vi "need_to_update_settings.vi"(1 "previous settings value cluster":T1, 2 "settings value cluster":T1) -> (0 "New Settings Exist?":bool)   [LabVIEW 2015]
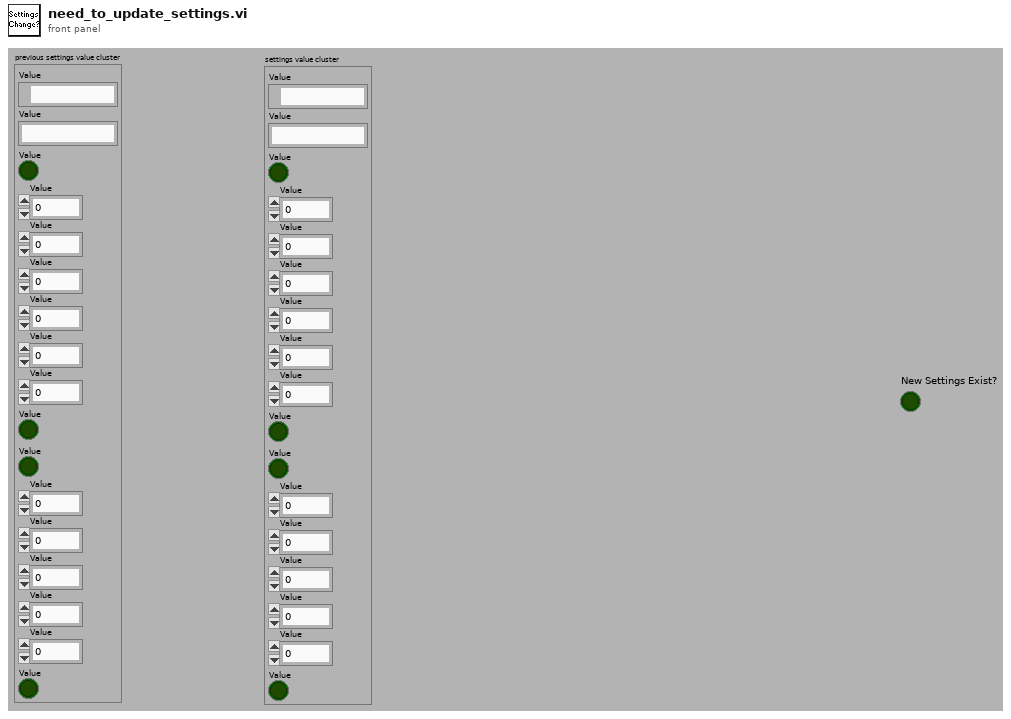
[diagram p1: front panel]
types:
  T1 = cluster{"Value":path, "Value":string, "Value":bool, "Value":dbl, "Value":dbl, "Value":i32, "Value":i32, "Value":dbl, "Value":u16, "Value":bool, "Value":bool, "Value":i32, "Value":i32, "Value":i32, "Value":u32, "Value":i32, "Value":bool}
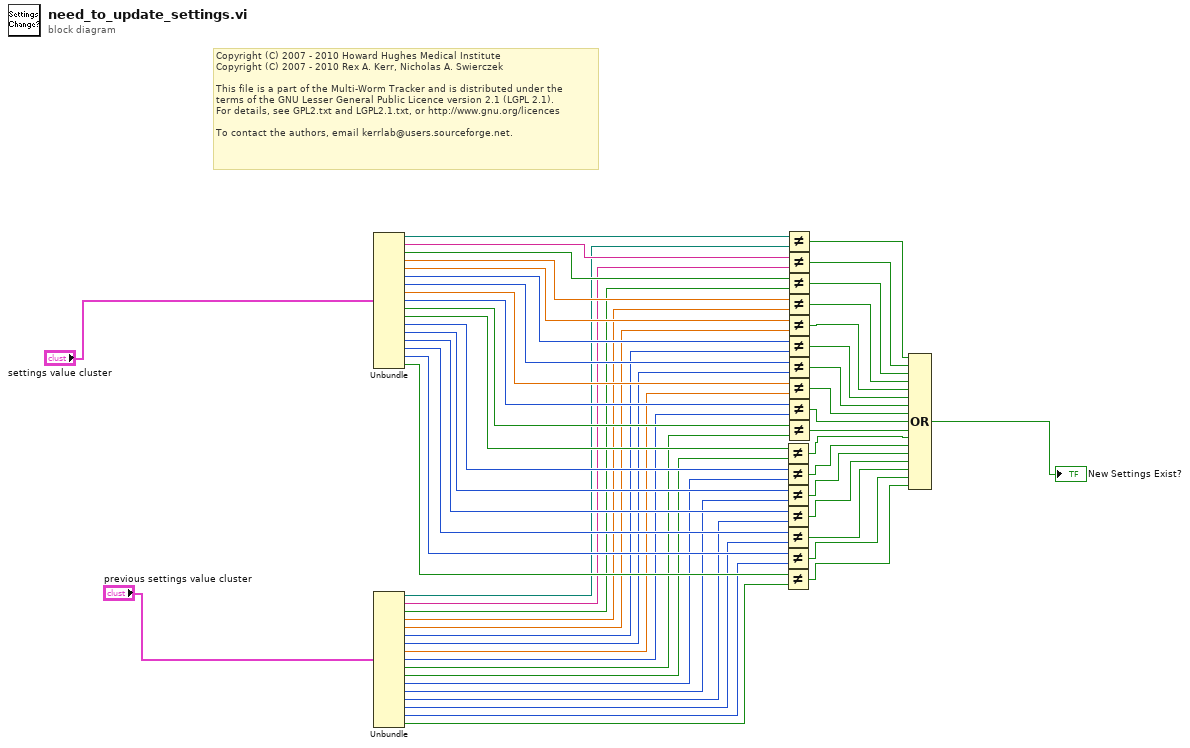
[diagram p0: block diagram]
diagram:
  # "Copyright (C) 2007 - 2010 Howard Hughes Medical Institute\nCopyright (C) 2007 - 2010 Rex A. Kerr, Nicholas A. Swierczek\n \nThis file is a part of the Multi-Worm Tracker and is distributed under the\nterms of the GNU Lesser General Public Licence version 2.1 (LGPL 2.1).\nFor details, see GPL2.txt and LGPL2.1.txt, or http://www.gnu.org/licences\n \nTo contact the authors, email kerrlab@users.sourceforge.net."
  n1 = Unbundle("settings value cluster") -> ("Value"=w52:path, "Value"=w51:string, "Value"=w50:bool, "Value"=w49:dbl, "Value"=w48:dbl, "Value"=w47:i32, "Value"=w46:i32, "Value"=w45:dbl, "Value"=w44:u16, "Value"=w43:bool, "Value"=w42:bool, "Value"=w41:i32, "Value"=w40:i32, "Value"=w39:i32, "Value"=w38:u32, "Value"=w37:i32, "Value"=w36:bool)
  n2 = Unbundle("previous settings value cluster") -> ("Value"=w35:path, "Value"=w34:string, "Value"=w33:bool, "Value"=w32:dbl, "Value"=w31:dbl, "Value"=w30:i32, "Value"=w29:i32, "Value"=w28:dbl, "Value"=w27:u16, "Value"=w26:bool, "Value"=w25:bool, "Value"=w24:i32, "Value"=w23:i32, "Value"=w22:i32, "Value"=w21:u32, "Value"=w20:i32, "Value"=w19:bool)
  n3 = Not Equal?(x=w42, y=w25) -> (x != y?=w7:bool)
  n4 = Not Equal?(x=w41, y=w24) -> (x != y?=w6:bool)
  n5 = Not Equal?(x=w40, y=w23) -> (x != y?=w5:bool)
  n6 = Not Equal?(x=w39, y=w22) -> (x != y?=w4:bool)
  n7 = Not Equal?(x=w38, y=w21) -> (x != y?=w3:bool)
  n8 = Not Equal?(x=w37, y=w20) -> (x != y?=w2:bool)
  n9 = Not Equal?(x=w36, y=w19) -> (x != y?=w1:bool)
  n10 = Not Equal?(x=w52, y=w35) -> (x != y?=w17:bool)
  n11 = Not Equal?(x=w51, y=w34) -> (x != y?=w16:bool)
  n12 = Not Equal?(x=w50, y=w33) -> (x != y?=w15:bool)
  n13 = Not Equal?(x=w49, y=w32) -> (x != y?=w14:bool)
  n14 = Not Equal?(x=w48, y=w31) -> (x != y?=w13:bool)
  n15 = Not Equal?(x=w47, y=w30) -> (x != y?=w12:bool)
  n16 = Not Equal?(x=w46, y=w29) -> (x != y?=w11:bool)
  n17 = Not Equal?(x=w45, y=w28) -> (x != y?=w10:bool)
  n18 = Not Equal?(x=w44, y=w27) -> (x != y?=w9:bool)
  n19 = Not Equal?(x=w43, y=w26) -> (x != y?=w8:bool)
  n20 = Compound Arithmetic op=OR(w17, w16, w15, w14, w13, w12, w11, w10, w9, w8, w7, w6, w5, w4, w3, w2, w1) -> (→"New Settings Exist?":bool)
